vi "setUp.vi"(8 "error in (no error)":errorcluster, 11 "reference in":refnum<class "Test TCP Stream Transmission.lvclass">) -> (0 "error out":errorcluster, 3 "reference out":refnum<class "Test TCP Stream Transmission.lvclass">)   [LabVIEW 2020, in "Test TCP Stream Transmission.lvclass"]
doc: "setUp runs prior to the test method during test execution. Use this method to initialize any object data required by your tests."
uses:
  Test TCP Stream Transmission.lvclass
  <vilib>/addons/_JKI Toolkits/VI Tester/TestCase.llb/TestCase.lvclass
  Source/Protocols/TCP Strategy/TCP Stream Initiator/TCP Stream Initiator.lvclass
  Source/Ciphers/AES/AES.lvclass
  Source/Ciphers/AES/Ton Plomp Encryption/AES-Modes.ctl
  Source/Ciphers/AES/Ton Plomp Encryption/Encryption.lvlib
  Source/Abstract Classes/Message Stream/Message Stream.lvclass
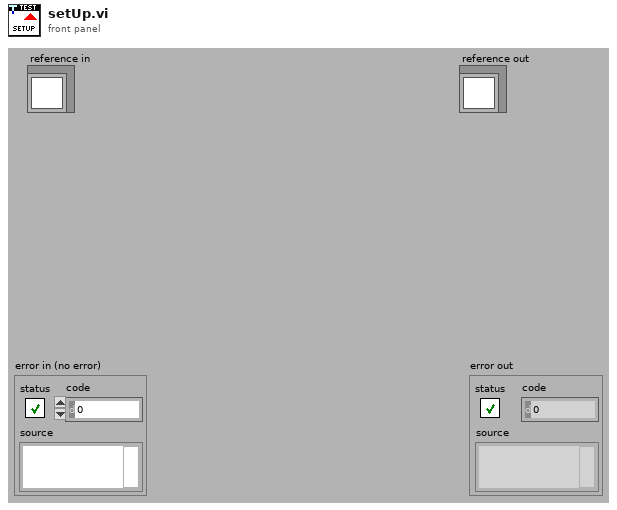
[diagram p1: front panel]
types:
  T1 = typedef "Encryption.lvlib/AES-Modes.ctl" = enum16{"ECB", "CBC", "CFB128", "OFB"}
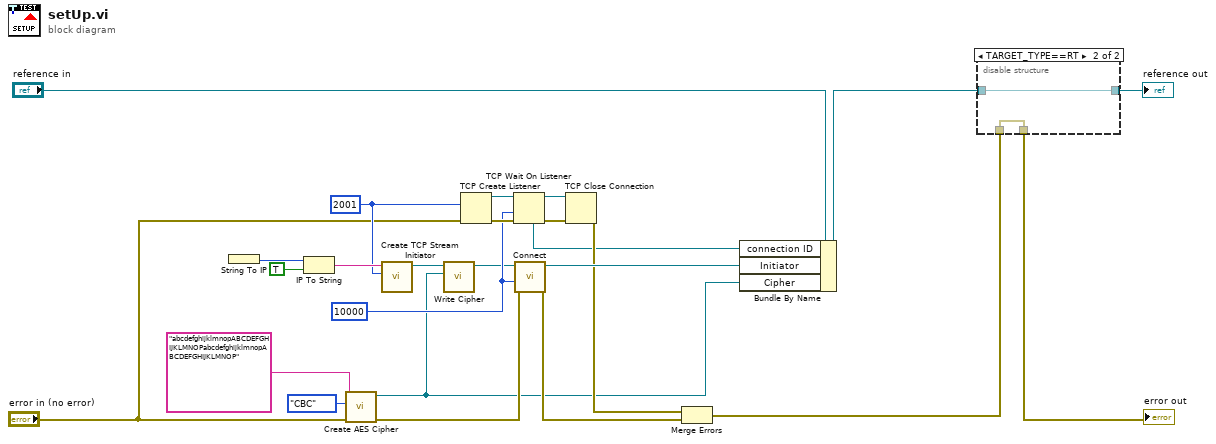
[diagram p0: block diagram]
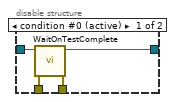
[diagram p2: hidden frame]
diagram:
  w15 = u16 2001 ("port")
  w19 = 10000 ("timeout")
  n1 = String To IP() -> (0:w17:u32)  [unwired: 1 in]
  n2 = IP To String(1:TRUE ("dot notation? (F)"), 2:w17) -> (0:w16:string)
  n3 = call "Create AES Cipher.vi"("error in (no error)"="error in (no error)", "Operation Mode"=AES-Modes."CBC", "Cipher Key"="abcdefghijklmnopABCDEFGHIJKLMNOPabcdefghijklmnopABCDEFGHIJKLMNOP") -> ("error out"=w2:errorcluster, "AES out"=w1:refnum<class "AES.lvclass">)  [unwired: 7 in]
  n4 = call "Create TCP Stream Initiator.vi"("Remote Port"=w15, "Remote Address"=w16) -> ("TCP Stream Initiator"=w5:refnum<class "TCP Stream Initiator.lvclass">)  [unwired: 9 in]
  n5 = call "Write Cipher.vi"("Cipher"=w1, "Message Stream in"=w5) -> ("Message Stream out"=w4:refnum<class "TCP Stream Initiator.lvclass">)  [unwired: 9 in]
  n6 = TCP Create Listener(8:"error in (no error)", 10:w15) -> (0:w23:errorcluster, 3:w22:refnum<k5>)  [unwired: 3 in, 1 out]
  n7 = TCP Wait On Listener(8:w23, 9:w19, 11:w22) -> (0:w21:errorcluster, 3:w20:refnum<k5>, 4:w11:refnum<k5>)  [unwired: 1 in, 2 out]
  n8 = call-dynamic "Connect.vi"("error in (no error)"=w2, "timeout"=w19, "TCP Stream Initiator in"=w4) -> ("error out"=w13:errorcluster, "TCP Stream Initiator out"=w14:refnum<class "TCP Stream Initiator.lvclass">)  [unwired: 7 in]
  n9 = TCP Close Connection(connection ID=w20, error in (no error)=w21) -> (error out=w12:errorcluster)  [unwired: 1 in, 1 out]
  n10 = Merge Errors(w12, w13) -> (w10:errorcluster)
  n11 = Bundle By Name(cluster="reference in", "connection ID"=w11, "Initiator"=w14, "Cipher"=w1) -> (w8:refnum<class "Test TCP Stream Transmission.lvclass">)
  n12 = disable-structure shown="TARGET_TYPE==RT" {
    disable-tunnel: w10 -> [w29 w30]
    disable-tunnel: [w28 w30] -> w25
    disable-tunnel: [w27 w31] -> w24
    disable-tunnel: w8 -> [w26 w31]
    frame condition #0 (active) {
      n13 = call <vilib>:"WaitOnTestComplete.vi"("error in (no error)"=w29, "TestCase in"=w26) -> ("error out"=w28:errorcluster, "TestCase out"=w27:refnum<class "Test TCP Stream Transmission.lvclass">)  [unwired: 8 in]
    }
    frame condition #1 {
    }
  }
  "error out" <- w25
  "reference out" <- w24
